vi "Macro Learn.vi"(0 "VISA resource name":refnum<visa-resource-name>, 5 "Learn (F: Off)":bool, 11 "error in (no error)":errorcluster) -> (4 "VISA resource name out":refnum<visa-resource-name>, 15 "error out":errorcluster)   [LabVIEW 2012, in "NH Research Regenerative Test Series.lvlib"]
doc: "This command sets the macro learn mode state. If learn mode is TRUE, the following commands will be recorded and NOT executed:\n\nReset Measurements.vi\nInitiate Measurement.vi\nInitiate Measurement Trigger.vi\nMacro Wait Time.vi\nMacro Wait Slew.vi\nMacro Wait Trigger.vi\nSet Output Operation State.vi\nConfigure Slew Rate.vi\n\n Set learn mode to FALSE to stop recording commands (normal operation)."
uses:
  <instrlib>/NH Research Regenerative Test Series/NH Research Regenerative Test Series.lvlib
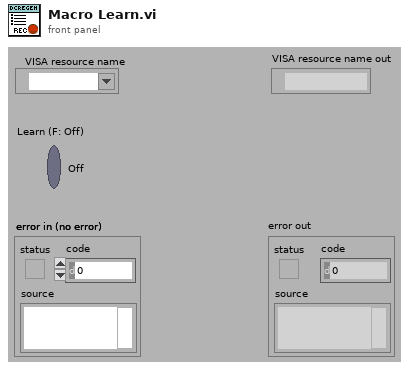
[diagram p1: front panel]
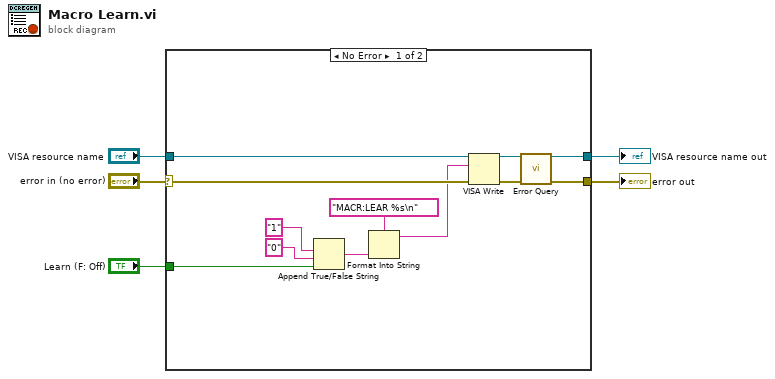
[diagram p0: block diagram]
diagram:
  n1 = case shown="No Error" "error in (no error)" {
    selector: "error in (no error)" -> [w9 w19]
    tunnel: "VISA resource name" -> [w17 w18]
    tunnel: [w16 w18] -> w4
    tunnel: [w15 w19] -> w3
    tunnel: "Learn (F: Off)" -> [w10 _]
    frame No Error {
      n2 = Append True/False String(1:w10, 2:"0", 3:"1") -> (0:w7:string)  [unwired: 1 in]
      n3 = Format Into String(format string="MACR:LEAR %s\n", w7) -> (resulting string=w6:string)  [unwired: 2 in, 1 out]
      n4 = VISA Write(VISA resource name=w17, write buffer=w6, error in (no error)=w9) -> (VISA resource name out=w14:refnum<visa-resource-name>, error out=w13:errorcluster)  [unwired: 1 out]
      n5 = call <instrlib>:"Error Query.vi"("VISA resource name"=w14, "error in (no error)"=w13) -> ("VISA resource name out"=w16:refnum<visa-resource-name>, "error out"=w15:errorcluster)  [unwired: 10 in, 2 out]
    }
    frame Error {
    }
  }
  "error out" <- w3
  "VISA resource name out" <- w4
